vi "VAT_valve_get_software_version.vi"(0 "VAT Valve COM port":refnum<visa-resource-name>, 11 "error in (no error)":errorcluster) -> (4 "VAT Valve COM port out":refnum<visa-resource-name>, 13 "Software Version":dbl, 15 "error out":errorcluster)   [LabVIEW 2019]
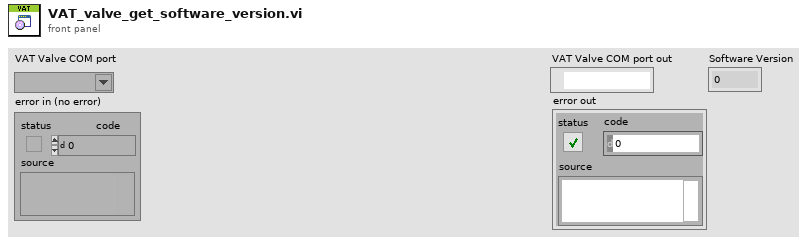
[diagram p1: front panel]
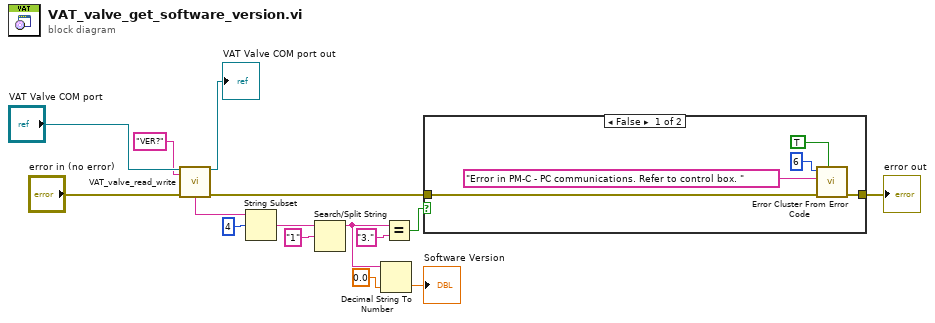
[diagram p0: block diagram]
diagram:
  n1 = call "VAT_valve_read_write.vi"("VAT Valve COM port"="VAT Valve COM port", "Write String"="VER?", "error in (no error)"="error in (no error)") -> ("VAT Valve COM port out"=→"VAT Valve COM port out":refnum<visa-resource-name>, "Read String"=w2:string, "error out"=w5:errorcluster)  [unwired: 10 in]
  n2 = String Subset(string=w2, offset (0)=4) -> (substring=w15:string)  [unwired: 1 in]
  n3 = Search/Split String(string=w15, search string/char (-)="1") -> (substring before match=w9:string)  [unwired: 1 in, 2 out]
  n4 = Decimal String To Number(string=w9, default (0L)=0.0) -> (number=→"Software Version":dbl)  [unwired: 1 in, 1 out]
  n5 = Equal?(x=w9, y="3.") -> (x = y?=w11:bool)
  n6 = case shown="False" w11 {
    tunnel: [w17 w21] -> w10
    tunnel: w5 -> [w16 w21]
    frame False {
      n7 = call <vilib>:"Error Cluster From Error Code.vi"("show call chain? (False)"=TRUE, "error in (no error)"=w16, "error message (\"\")"="Error in PM-C - PC communications. Refer to control box. " ("error message (\"\")"), "error code (0)"=6) -> ("error out"=w17:errorcluster)  [unwired: 5 in]
    }
    frame True {
    }
  }
  "error out" <- w10
